vi "library_variable.vi"() -> ()   [LabVIEW 2020, in "core.lvlib" / "core_data.lvlib"]
uses:
  core_data.lvlib
  core_data.ctl
  tour_in_progress.ctl
  chessboard_index.ctl
  chess_square.ctl
  neighbour_square.ctl
panel:
  in  "core_data":refnum<data-value>
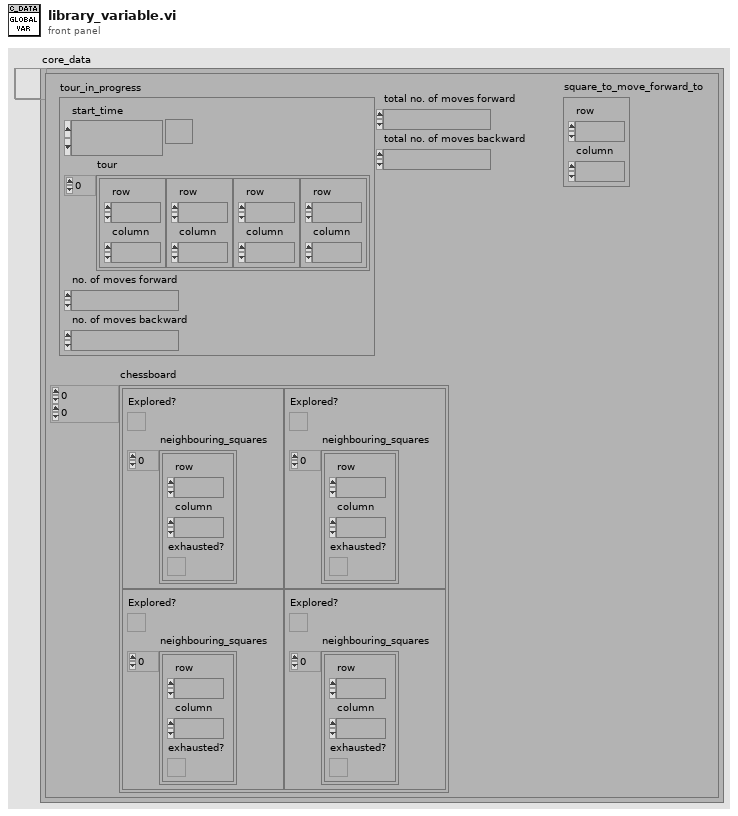
[diagram p1: front panel]
diagram:
